vi "MISC Get Path Information.vi"(11 "Error In (no error)":errorcluster) -> (3 "Top Level VI Name":string, 4 "Root Drive":path, 6 "Application Directory":path, 8 "Support Directory":path, 10 "Top Level VI Path":path, 14 "Development Environment":bool, 15 "Error Out":errorcluster)   [LabVIEW 2012]
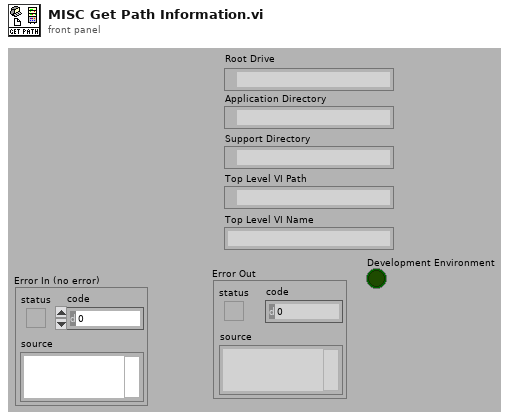
[diagram p1: front panel]
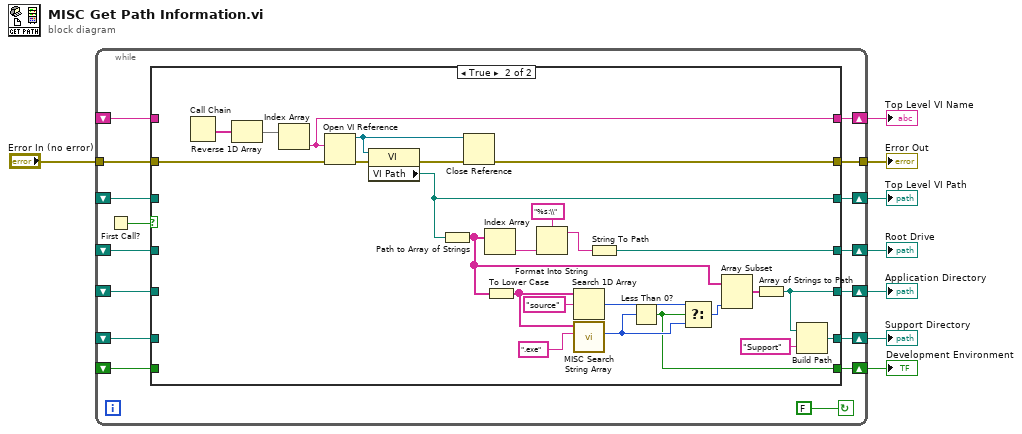
[diagram p0: block diagram]
diagram:
  n1 = while {
    tunnel: "Error In (no error)" -> [w24]
    tunnel: [w23] -> w7
    shift-right: [w17] -> w3
    shift-left: _ -> [w12]
    shift-right: [w18] -> w4
    shift-left: _ -> [w13]
    shift-right: [w19] -> w5
    shift-left: _ -> [w14]
    shift-right: [w20] -> w6
    shift-left: _ -> [w15]
    shift-right: [w21] -> w2
    shift-left: _ -> [w16]
    shift-right: [w10] -> w1
    shift-left: _ -> [w9]
    stop <- FALSE continue-if-true
    n2 = First Call?() -> (First Call?: T/F=w22:bool)
    n3 = case shown="True" w22 {
      tunnel: [w28 w56] -> w19
      tunnel: [w31 w53] -> w21
      tunnel: w24 -> [w29 w49]
      tunnel: [w29 w48] -> w23
      tunnel: [w27 w46] -> w18
      tunnel: [w26 w44] -> w17
      tunnel: [w30 w43] -> w20
      tunnel: w16 -> [w31 _]
      tunnel: w15 -> [w30 _]
      tunnel: w14 -> [w28 _]
      tunnel: w13 -> [w27 _]
      tunnel: w12 -> [w26 _]
      tunnel: [w25 w32] -> w10
      tunnel: w9 -> [w25 _]
      frame False {
      }
      frame True {
        n4 = Call Chain() -> (call chain=w55:string[])
        n5 = Reverse 1D Array(array=w55) -> (reversed array=w54:string[])
        n6 = Index Array(array=w54) -> (element=w53:string)  [unwired: 1 in]
        n7 = Open VI Reference(vi path=w53, error in (no error)=w49) -> (vi reference=w50:refnum<vi>, error out=w52:errorcluster)  [unwired: 4 out]
        n8 = property class="VI"(reference=w50, error in=w52) -> (error out=w51:errorcluster, "VI Path"=w43:path)  [unwired: 1 out]
        n9 = Path to Array of Strings(0:w43) -> (2:w42:string[])  [unwired: 1 out]
        n10 = Close Reference(reference=w50, error in (no error)=w51) -> (error out=w48:errorcluster)
        n11 = Index Array(array=w42) -> (element=w34:string)  [unwired: 1 in]
        n12 = To Lower Case(string=w42) -> (all lower case string=w40:string[])
        n13 = Format Into String(format string="%s:\\", w34) -> (resulting string=w33:string)  [unwired: 2 in, 1 out]
        n14 = Search 1D Array(1D array=w40, element="source") -> (index of element=w37:i32)  [unwired: 1 out]
        n15 = call "MISC Search String Array.vi"("String"=".exe" ("element"), "String Array"=w40) -> ("First Index"=w36:i32)  [unwired: 1 in, 8 out]
        n16 = String To Path(string=w33) -> (path=w56:path)
        n17 = Less Than 0?(x=w36) -> (x < 0?=w32:bool)
        n18 = Select(t=w37, s=w32, f=w36) -> (s? t:f=w38:i32)
        n19 = Array Subset(array=w42, length=w38) -> (w47:string[])  [unwired: 1 in]
        n20 = Array of Strings to Path(0:w47) -> (2:w46:path)  [unwired: 1 out]
        n21 = Build Path(base path=w46, name or relative path="Support") -> (appended path=w44:path)
      }
    }
  }
  "Root Drive" <- w5
  "Error Out" <- w7
  "Top Level VI Name" <- w2
  "Top Level VI Path" <- w6
  "Application Directory" <- w4
  "Support Directory" <- w3
  "Development Environment" <- w1
